vi "Trigger Response Notifier.vi"(8 "error in (no error)":errorcluster, 10 "Response String in":string, 11 "Return Request in":T1) -> (0 "error out":errorcluster)   [LabVIEW 2017, in "SSH.lvlib"]
uses:
  SSH.lvlib
  Return Request Configuration.ctl
  Response Configuration.ctl
  Expected Response String Config.ctl
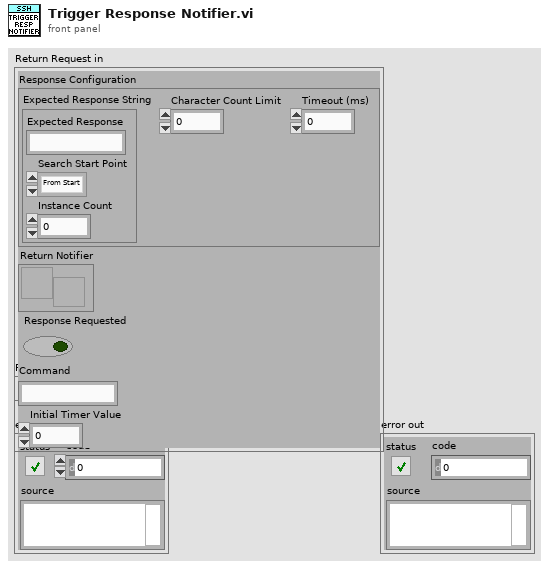
[diagram p1: front panel]
types:
  T1 = typedef "SSH.lvlib/Return Request Configuration.ctl" = cluster{"Response Configuration":T2, "Return Notifier":refnum<notifier>, "Response Requested":bool, "Command":string, "Initial Timer Value":u32}
  T2 = typedef "SSH.lvlib/Response Configuration.ctl" = cluster{"Expected Response String":T3, "Character Count Limit":i32, "Timeout (ms)":i32}
  T3 = typedef "SSH.lvlib/Expected Response String Config.ctl" = cluster{"Expected Response":string, "Search Start Point":enum16{"From Start", "From End"}, "Instance Count":i32}
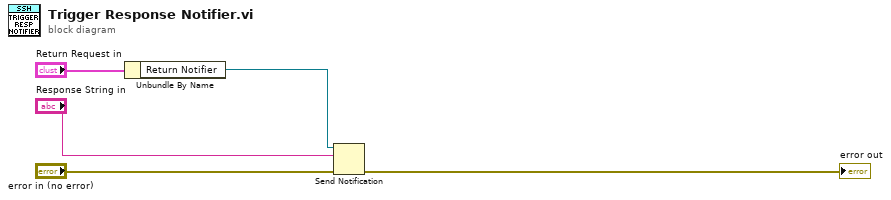
[diagram p0: block diagram]
diagram:
  n1 = Unbundle By Name("Return Request in") -> ("Return Notifier"=w2:refnum<notifier>)
  n2 = Send Notification(notification="Response String in", notifier=w2, error in (no error)="error in (no error)") -> (error out=→"error out":errorcluster)  [unwired: 1 out]
